vi "Convert to Field  Orientation.vi"(7 "Compass Heading":T4 scale format="%.3f", 11 "Direction in":T1 {"Rotate(Yaw) CCW 1 CW -1" scale=1.0..-1.0; "Traverse"."Angle" scale format="%.3f"; "Traverse"."Velocity" scale=-1.0..1.0 scale format="%.1f"}) -> (3 "Corrected Direction out":T1 {"Rotate(Yaw) CCW 1 CW -1" scale=1.0..-1.0; "Traverse"."Angle" scale format="%.3f"; "Traverse"."Velocity" scale=-1.0..1.0 scale format="%.1f"})   [LabVIEW 2023, in "Thor-SwerveDrive_ACT.lvlib"]
uses:
  Thor-SwerveDrive_ACT.lvlib
  Shared Code/TypeDefs/Dial_Compase heading unit circle CCW positive.ctl
  Shared Code/TypeDefs/Level_Velocity plus-minus 1.ctl
  Shared Code/TypeDefs/Cluster_Module Velocity-Direction-Rotations.ctl
  Shared Code/TypeDefs/Cluster_CMD_Direction Data.ctl
  Type Defs/NUM_Rotate Input.ctl
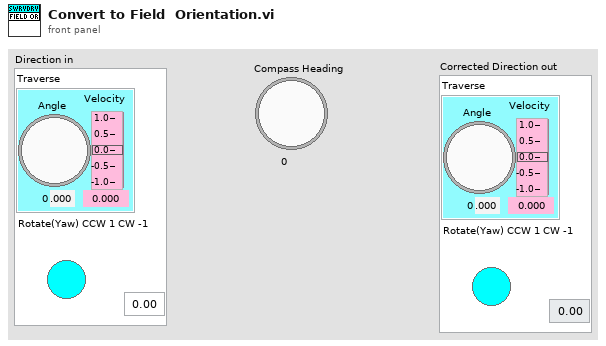
[diagram p1: front panel]
types:
  T1 = typedef "Cluster_CMD_Direction Data.ctl" = cluster{"Traverse":T2, "Rotate(Yaw) CCW 1 CW -1":T5}
  T2 = typedef "Cluster_Module Velocity-Direction-Rotations.ctl" = cluster{"Velocity":T3, "Angle":T4, "Rotations Count":dbl}
  T3 = typedef "Level_Velocity plus-minus 1.ctl" = dbl
  T4 = typedef "Dial_Compase heading unit circle CCW positive.ctl" = dbl
  T5 = typedef "NUM_Rotate Input.ctl" = dbl
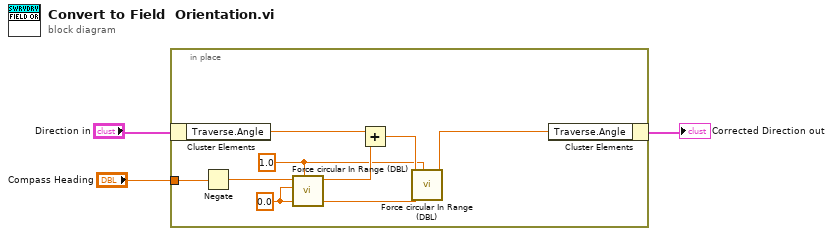
[diagram p0: block diagram]
diagram:
  n1 = in-place {
    in-place-border: "Compass Heading" -> [w11]
    w5 = 0.0 ("Max")
    w6 = 1.0 ("Max")
    n2 = in-place-cluster #1("Direction in") -> ("Traverse.Angle"=w9:T4)
    n3 = Negate(x=w11) -> (-x=w10:T4)
    n4 = call "Force circular In Range (DBL).vi"("Max"=w6, "Min"=w5, "Value"=w10) -> ("Value Out"=w8:dbl)  [unwired: 7 in, 1 out]
    n5 = Add(x=w9, y=w8) -> (x+y=w7:T4)
    n6 = call "Force circular In Range (DBL).vi"("Max"=w6, "Min"=w5, "Value"=w7) -> ("Value Out"=w4:dbl)  [unwired: 7 in, 1 out]
    n7 = in-place-cluster #1("Traverse.Angle"=w4) -> (→"Corrected Direction out":T1)
  }
